vi "Validate_Rect.vi"(1 "rect":T1) -> (0 "valid":bool)   [LabVIEW 2012]
doc: "Returns true if specified rect encloses non-zero area"
uses:
  <userlib>/BIAS2/subvis/ROI_rect.ctl
panel:
  # "Validates rect by checking it has non-zero area"
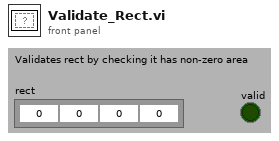
[diagram p1: front panel]
types:
  T1 = typedef "ROI_rect.ctl" = cluster{"left":i32, "top":i32, "right":i32, "bottom":i32}
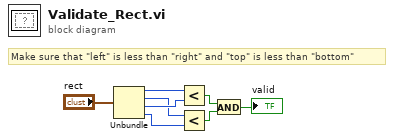
[diagram p0: block diagram]
diagram:
  # "Make sure that \"left\" is less than \"right\" and \"top\" is less than \"bottom\""
  n1 = Unbundle("rect") -> ("left"=w7:i32, "top"=w5:i32, "right"=w6:i32, "bottom"=w4:i32)
  n2 = Less?(x=w7, y=w6) -> (x < y?=w3:bool)
  n3 = Less?(x=w5, y=w4) -> (x < y?=w2:bool)
  n4 = And(x=w3, y=w2) -> (x .and. y?=→"valid":bool)
